vi "Destroy Events.vi"(0 "Display State In":T1={"Prompt"="Click to add", "Listbox"=refnum, "events"={"Items Changed"=refnum, "List Changed"=refnum}}, 9 "Container State":T3, 11 "error in (no error)":errorcluster) -> (4 "Display State Out":T1={"Prompt"="Click to add", "Listbox"=refnum, "events"={"Items Changed"=refnum, "List Changed"=refnum}}, 15 "error out":errorcluster)   [LabVIEW 2020, in "KListbox.xctl"]
uses:
  <vilib>/_xctls/Container State.ctl
  KListbox.xctl
  <vilib>/_xctls/XControlSupport.lvlib
  Event Action.ctl
  Events.ctl
  State.ctl
panel:
  # "Add Controls & Indicators that form the parameters of the method here. Hook them to the connector pane. Do not delete the controls & indicators that are already hooked to the connector pane.\n \nTo setup the parameters  for this method, right click on this item in the Project Tree & select \"Configure Method...\"."
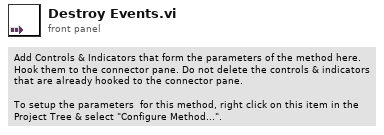
[diagram p1: front panel]
types:
  T1 = typedef "KListbox.xctl/State.ctl" = cluster{"Prompt":string, "Listbox":refnum<vi>, "events":T2}
  T2 = typedef "KListbox.xctl/Events.ctl" = cluster{"Items Changed":refnum<user-event>, "List Changed":refnum<user-event>}
  T3 = typedef "XControlSupport.lvlib/Container State.ctl" = cluster{"Indicator?":bool, "Run Mode?":bool, " Refnum":refnum<vi>}
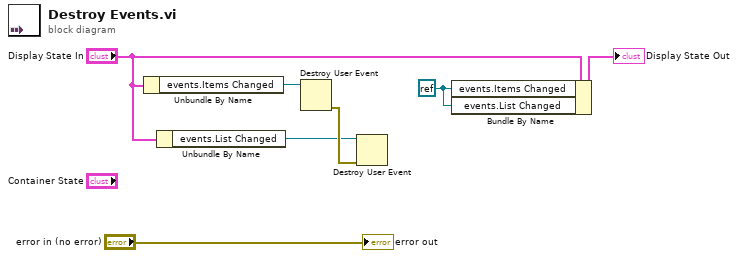
[diagram p0: block diagram]
diagram:
  w1 = refnum<k0> refnum
  n1 = Unbundle By Name("Display State In") -> ("events.Items Changed"=w6:refnum<user-event>)
  n2 = Unbundle By Name("Display State In") -> ("events.List Changed"=w3:refnum<user-event>)
  n3 = Destroy User Event(user event=w6) -> (error out=w4:errorcluster)  [unwired: 1 in]
  n4 = Destroy User Event(user event=w3, error in=w4) -> ()  [unwired: 1 out]
  n5 = Bundle By Name(cluster="Display State In", "events.Items Changed"=w1, "events.List Changed"=w1) -> (→"Display State Out":T1)
  "error out" <- "error in (no error)"
